vi "Tools_KeyedArray Values.vi"(7 "array in":T1) -> (2 "values":string[](array[string]), 3 "duplicate array":T1)   [LabVIEW 2011]
doc: "Returns an array containing the values of all the elements in <B>array in</B>."
uses:
  Tools_KeyedArray KeyedArray.ctl
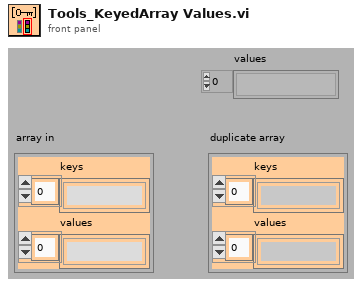
[diagram p1: front panel]
types:
  T1 = typedef "Tools_KeyedArray KeyedArray.ctl" = cluster{"keys":string[], "values":string[]}
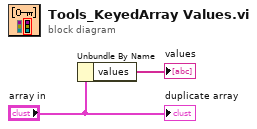
[diagram p0: block diagram]
diagram:
  n1 = Unbundle By Name("array in") -> ("values"=→"values":string[])
  "duplicate array" <- "array in"
